vi "CytecRead.vi"(5 "VISA resource name":refnum<visa-resource-name>) -> (0 "error out":errorcluster, 1 "SwitchMatrix":bool[][](array[boolean]), 2 "VISA resource name out":refnum<visa-resource-name>)   [LabVIEW 2021]
panel:
  in  "error in (no error)":errorcluster
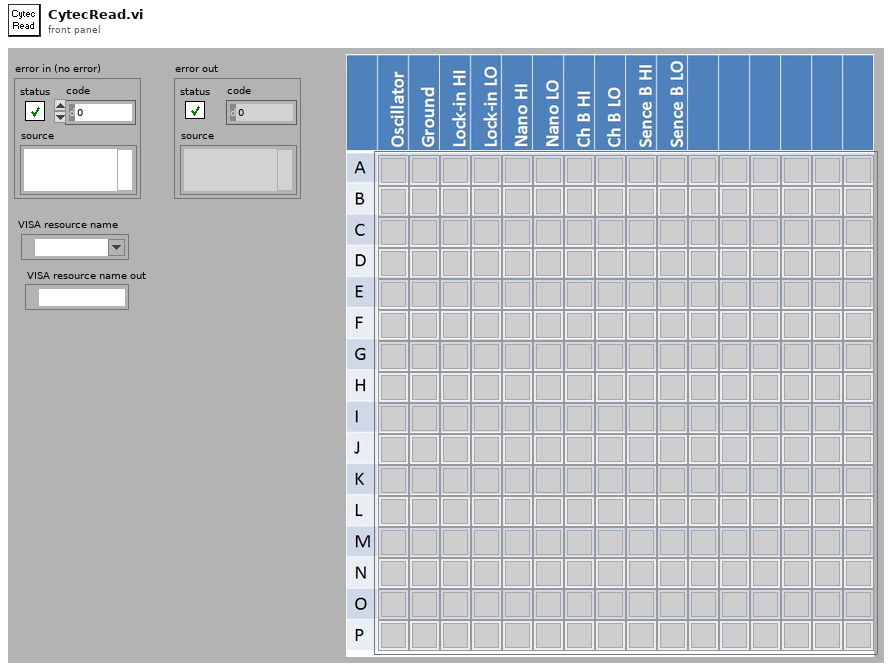
[diagram p1: front panel]
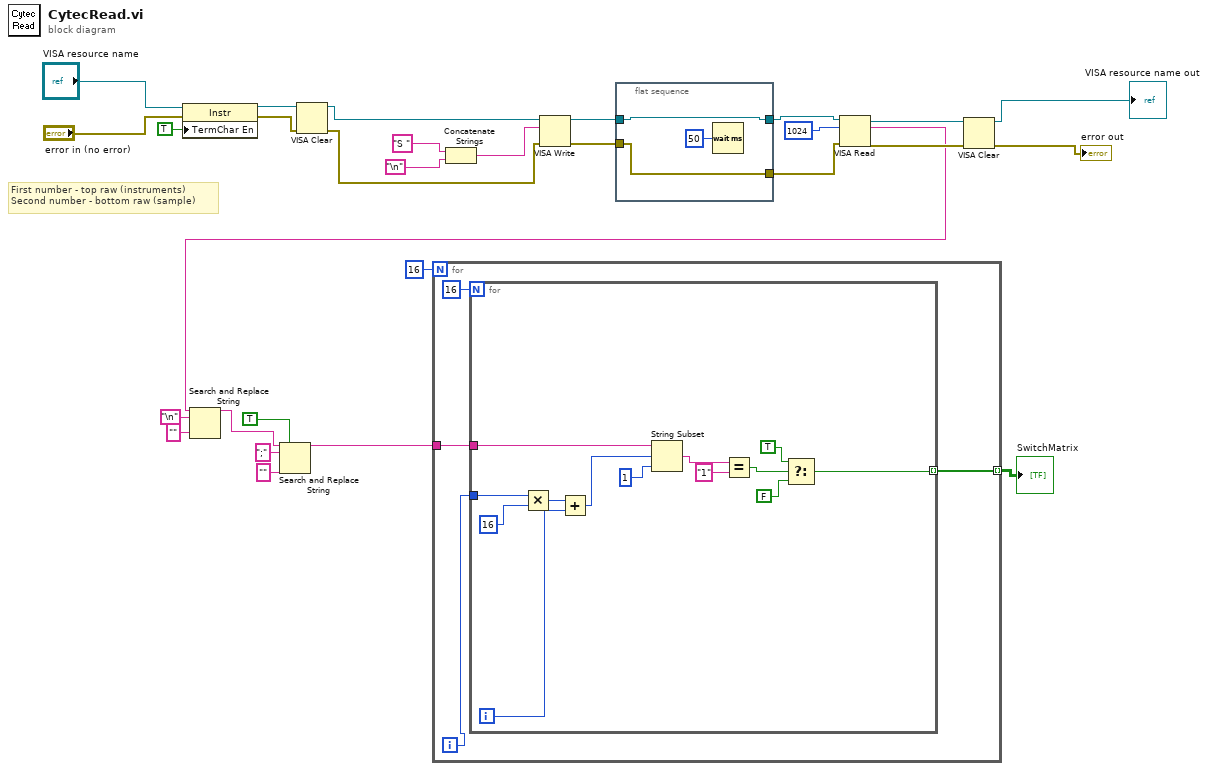
[diagram p0: block diagram]
diagram:
  # "First number - top raw (instruments)\nSecond number - bottom raw (sample)"
  n1 = property class="Instr"(reference="VISA resource name", error in="error in (no error)", "TermChar En"=TRUE ("Message Based Settings:Termination Character Enable")) -> (reference out=w22:refnum<visa-resource-name>, error out=w21:errorcluster)
  n2 = VISA Clear(VISA resource name=w22, error in (no error)=w21) -> (VISA resource name out=w20:refnum<visa-resource-name>, error out=w19:errorcluster)
  n3 = Concatenate Strings("S ", "\n") -> (w28:string)
  n4 = VISA Write(VISA resource name=w20, write buffer=w28, error in (no error)=w19) -> (VISA resource name out=w18:refnum<visa-resource-name>, error out=w17:errorcluster)  [unwired: 1 out]
  n5 = flat-sequence {
    tunnel: w18 -> [w31]
    tunnel: w17 -> [w30]
    tunnel: [w31] -> w16
    tunnel: [w30] -> w15
    frame #0 {
      n6 = Wait (ms)(milliseconds to wait=u32 50) -> ()  [unwired: 1 out]
    }
  }
  n7 = VISA Read(VISA resource name=w16, byte count=1024, error in (no error)=w15) -> (VISA resource name out=w14:refnum<visa-resource-name>, read buffer=w7:string, error out=w13:errorcluster)  [unwired: 1 out]
  n8 = Search and Replace String(input string=w7, search string="\n", replace string="" ("replace string (\"\")")) -> (result string=w4:string)  [unwired: 5 in, 3 out]
  n9 = Search and Replace String(replace all?=TRUE ("replace all? (F)"), input string=w4, search string=";", replace string="" ("replace string (\"\")")) -> (result string=w2:string)  [unwired: 4 in, 3 out]
  n10 = for {
    N: 16 -> [_]
    tunnel: w2 -> [w35]
    tunnel: [w33] -> w1 mode=indexing
    i -> [w34]
    n11 = for {
      N: 16 -> [_]
      tunnel: w35 -> [w49]
      tunnel: w34 -> [w48]
      tunnel: [w37] -> w33 mode=indexing
      i -> [w45]
      n12 = Multiply(x=w48, y=16) -> (x*y=w46:i32)
      n13 = Add(x=w46, y=w45) -> (x+y=w44:i32)
      n14 = String Subset(string=w49, offset (0)=w44, length (rest)=1 ("length (rest)")) -> (substring=w42:string)
      n15 = Equal?(x=w42, y="1") -> (x = y?=w40:bool)
      n16 = Select(t=TRUE, s=w40, f=FALSE) -> (s? t:f=w37:bool)
    }
  }
  "SwitchMatrix" <- w1
  n17 = VISA Clear(VISA resource name=w14, error in (no error)=w13) -> (VISA resource name out=→"VISA resource name out":refnum<visa-resource-name>, error out=→"error out":errorcluster)
